vi "playing with strings.vi"() -> ()   [LabVIEW 2018]
panel:
  out "Numeric 2":dbl
  out "String 3":string
  out "Numeric":dbl
  in  "String 2":string
  out "concatenated string":string
  in  "Array":string[][][](array[string])
  out "Boolean":bool
  in  "String":string
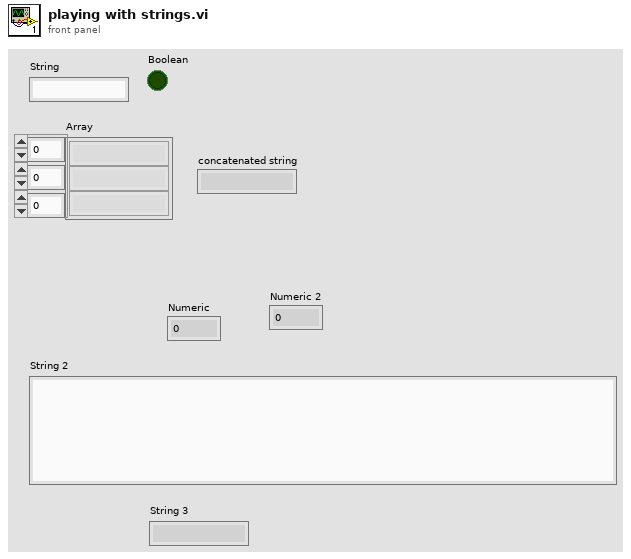
[diagram p1: front panel]
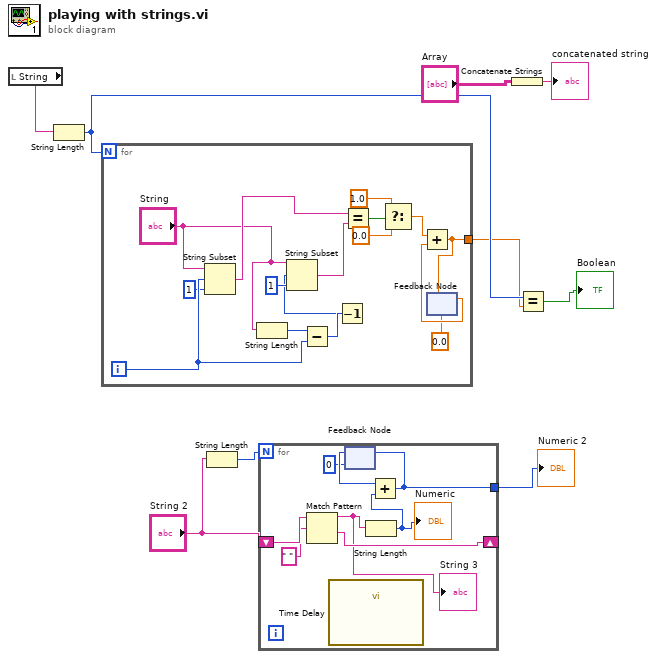
[diagram p0: block diagram]
diagram:
  n1 = local read "String"() -> (w9:string)
  n2 = String Length(string=w9) -> (length=w8:i32)
  n3 = for {
    N: w8 -> [_]
    tunnel: [w13] -> w7
    i -> [w24]
    n4 = String Subset(string="String", offset (0)=w24, length (rest)=1 ("length (rest)")) -> (substring=w21:string)
    n5 = String Length(string="String") -> (length=w25:i32)
    n6 = Subtract(x=w25, y=w24) -> (x-y=w11:i32)
    n7 = Decrement(x=w11) -> (x-1=w10:i32)
    n8 = String Subset(string="String", offset (0)=w10, length (rest)=1 ("length (rest)")) -> (substring=w20:string)
    n9 = Equal?(x=w21, y=w20) -> (x = y?=w19:bool)
    n10 = Select(t=1.0, s=w19, f=0.0) -> (s? t:f=w16:dbl)
    n11 = feedback #1(0.0) -> (w15:dbl)
    n12 = Add(x=w16, y=w15) -> (x+y=w13:dbl)
    n13 = feedback-in #1(w13) -> ()
  }
  n14 = String Length(string="String 2") -> (length=w2:i32)
  n15 = for {
    N: w2 -> [_]
    shift-right: [w31] -> _
    shift-left: "String 2" -> [w33]
    tunnel: [w26] -> w1
    n16 = Match Pattern(string=w33, regular expression=" ") -> (before substring=w30:string, after substring=w31:string)  [unwired: 1 in, 2 out]
    "String 3" <- w30
    n17 = call "Time Delay"() -> ()  [unwired: 11 in, 1 out]
    n18 = feedback #2(0) -> (w28:i32)
    n19 = String Length(string=w30) -> (length=w29:i32)
    "Numeric" <- w29
    n20 = Add(x=w28, y=w29) -> (x+y=w26:i32)
    n21 = feedback-in #2(w26) -> ()
  }
  "Numeric 2" <- w1
  n22 = Concatenate Strings("Array") -> (→"concatenated string":string)
  n23 = Equal?(x=w8, y=w7) -> (x = y?=→"Boolean":bool)
